vi "Calibration_Setup_file_2.0.vi"(2 "Data":T1={"Camera 1"={"Camera1"="", "Cam 1"=FALSE, "CAM1 Model"=enum."a2A5328-15ucBAS"}, "Camera 2"={"Camera2"="", "Cam 2"=FALSE, "CAM2 Model"=enum."a2A5328-15ucBAS"}, "Image"={"Camera1_Img"=refnum, "Camera2_Img"=refnum, "Img1_Orig_Disp"=refnum, "Img2_Orig_Disp"=refnum, "Img1_Orig_RGB"=refnum, "Img2_Orig_RGB"=refnum, "Blue_Plane_Extract"=refnum, "Subtracted_Plane"=refnum, "Img1_Binary"=refnum, "Img2_Binary"=refnum, "Crop_Mask"=refnum, "Img1_Save"=refnum, "Img2_Save"=refnum, "Img1_Cali_Full"=refnum, "Img2_Cali_Full"=refnum, "Img1_Cali_Detect"=refnum, "Img2_Cali_Detect"=refnum}, "Ques"={"Cam 1 queue"=refnum, "Cam 2 queue"=refnum, "Cam 1 - save queue"=refnum, "Cam 2 - save queue"=refnum, "Image Process Queue Size"=500, "Image Save Queue Size"=500, "Overload threshold"=500, "Max large object threshold"=0}, "Arduino SRS"={"Pinch-valve"="", "Actuator"=FALSE, "Open(T)/Close(F)"=FALSE}, "Pump"={"Pump"="", "Pump"=FALSE, "Pump State"=FALSE, "Pump Model"=enum."XLP6000", "Pump size"=FALSE, "Flush Size"=0, "Dispense Speed"=100, "Command"=""}, "Camera settings"={"Detection settings"={"Sample size threshold"=500, "Detection Region %"=30.0, "Timeout Sample"=200}, "Lens/camera settings"={"Aperture"=enum."Item 0", "Legacy Cam Attributes"=FALSE, "Max Framerate"=100, "Exposure Time"=1000.0, "Framerate"=15}, "Crop settings"={"Cam1"={"Rectangle 1"={"Left"=0, "Top"=0, "Right"=0, "Bottom"=0, "Rotation"=0.0}, "Camera Orientation 1"="", "Pixel to mm 1"=0.0}, "Cam2"={"Rectangle 2"={"Left"=0, "Top"=0, "Right"=0, "Bottom"=0, "Rotation"=0.0}, "Camera Orientation 2"="", "Pixel to mm 2"=0.0}}}, "Arduino ISS"={"Mega F3"="", "Phase3"=FALSE}, "Phase 3"={"Container nr."=0.0, "Mun. of containers"=0.0, "Size Interval"=0.0, "Initial size"=0.0, "Sorting sys."=FALSE, "Barcode"=""}, "Img_Capt"=FALSE, "Empty_Refill"=FALSE, "I don't think is in use"={"Crop"=FALSE, "Light intensity"=100, "Empty start"=1}, "Img_Capt Begin"=FALSE, "Extended setup"={"Location"="Station", "Latitude"="Station", "Longitude"="Station", "Determiner"="Station", "Sex"="Station", "Station"="", "Collection date"=""}, "Main interface"={"Sample Name"="Test Sample", "Operator"="JFR", "Species Name"="", "Other Notes"=""}, "Tap1"=0, "SystemVersion"=0, "System Serial"="", "Flush Insect"=FALSE, "Flush Error"=FALSE, "Start System"=FALSE, "Core JKI"={"Current VI Reference"=refnum, "Close Panel on Exit?"=FALSE}, "Calibration"={"Calibration 1"=path "C:/Users/au540322/Desktop/IHS_Project/images/Debris/Debris_0/Debris_0_2019_06_01-23-32-49-686.PNG", "Calibration 2"=path "C:/Users/au540322/Desktop/IHS_Project/images/Debris/Debris_0/Debris_0_2019_06_01-23-32-49-686.PNG", "Detect 1"=path "C:/Users/au540322/Desktop/IHS_Project/images/Debris/Debris_0/Debris_0_2019_06_01-23-32-49-686.PNG", "Detect 2"=path "C:/Users/au540322/Desktop/IHS_Project/images/Debris/Debris_0/Debris_0_2019_06_01-23-32-49-686.PNG"}} {"SystemVersion" items=["Standard", "XL"]; "Tap1" items=["Session Data", "Extended Setup", "Buffer", "Camera", "Dispenser", "Stats", "Connections"]; "I don't think is in use"."Empty start" min=1; "I don't think is in use"."Light intensity" scale=0.0..100.0; "Camera settings"."Crop settings"."Cam2"."Rectangle 2"."Rotation" format="%.2f"; "Camera settings"."Crop settings"."Cam2"."Rectangle 2"."Left" scale=0.0..1024.0; "Camera settings"."Crop settings"."Cam2"."Rectangle 2"."Right" scale=0.0..1024.0; "Camera settings"."Crop settings"."Cam1"."Rectangle 1"."Rotation" format="%.2f"; "Camera settings"."Crop settings"."Cam1"."Rectangle 1"."Left" scale=0.0..1024.0; "Camera settings"."Crop settings"."Cam1"."Rectangle 1"."Right" scale=0.0..1024.0; "Camera settings"."Lens/camera settings"."Framerate" min=1; "Camera settings"."Lens/camera settings"."Max Framerate" min=1; "Camera settings"."Detection settings"."Sample size threshold" min=1; "Pump"."Dispense Speed" min=1; "Pump"."Flush Size" min=0 max=6000 step=100; "Ques"."Overload threshold" min=1; "Ques"."Image Save Queue Size" min=1; "Ques"."Image Process Queue Size" min=1}, 3 "Path":string) -> ()   [LabVIEW 2024]
uses:
  controls/Data_JKI.ctl
  <vilib>/userDefined/High Color/IMAQdx.ctl
  <vilib>/vision/Image Controls.llb/IMAQ Image.ctl
  <vilib>/Utility/config.llb/Write Key (String).vi
  <vilib>/Utility/config.llb/NI_LVConfig.lvlib
panel:
  out "error out":errorcluster
  out "Error Out":errorcluster
  in  "Error In":errorcluster
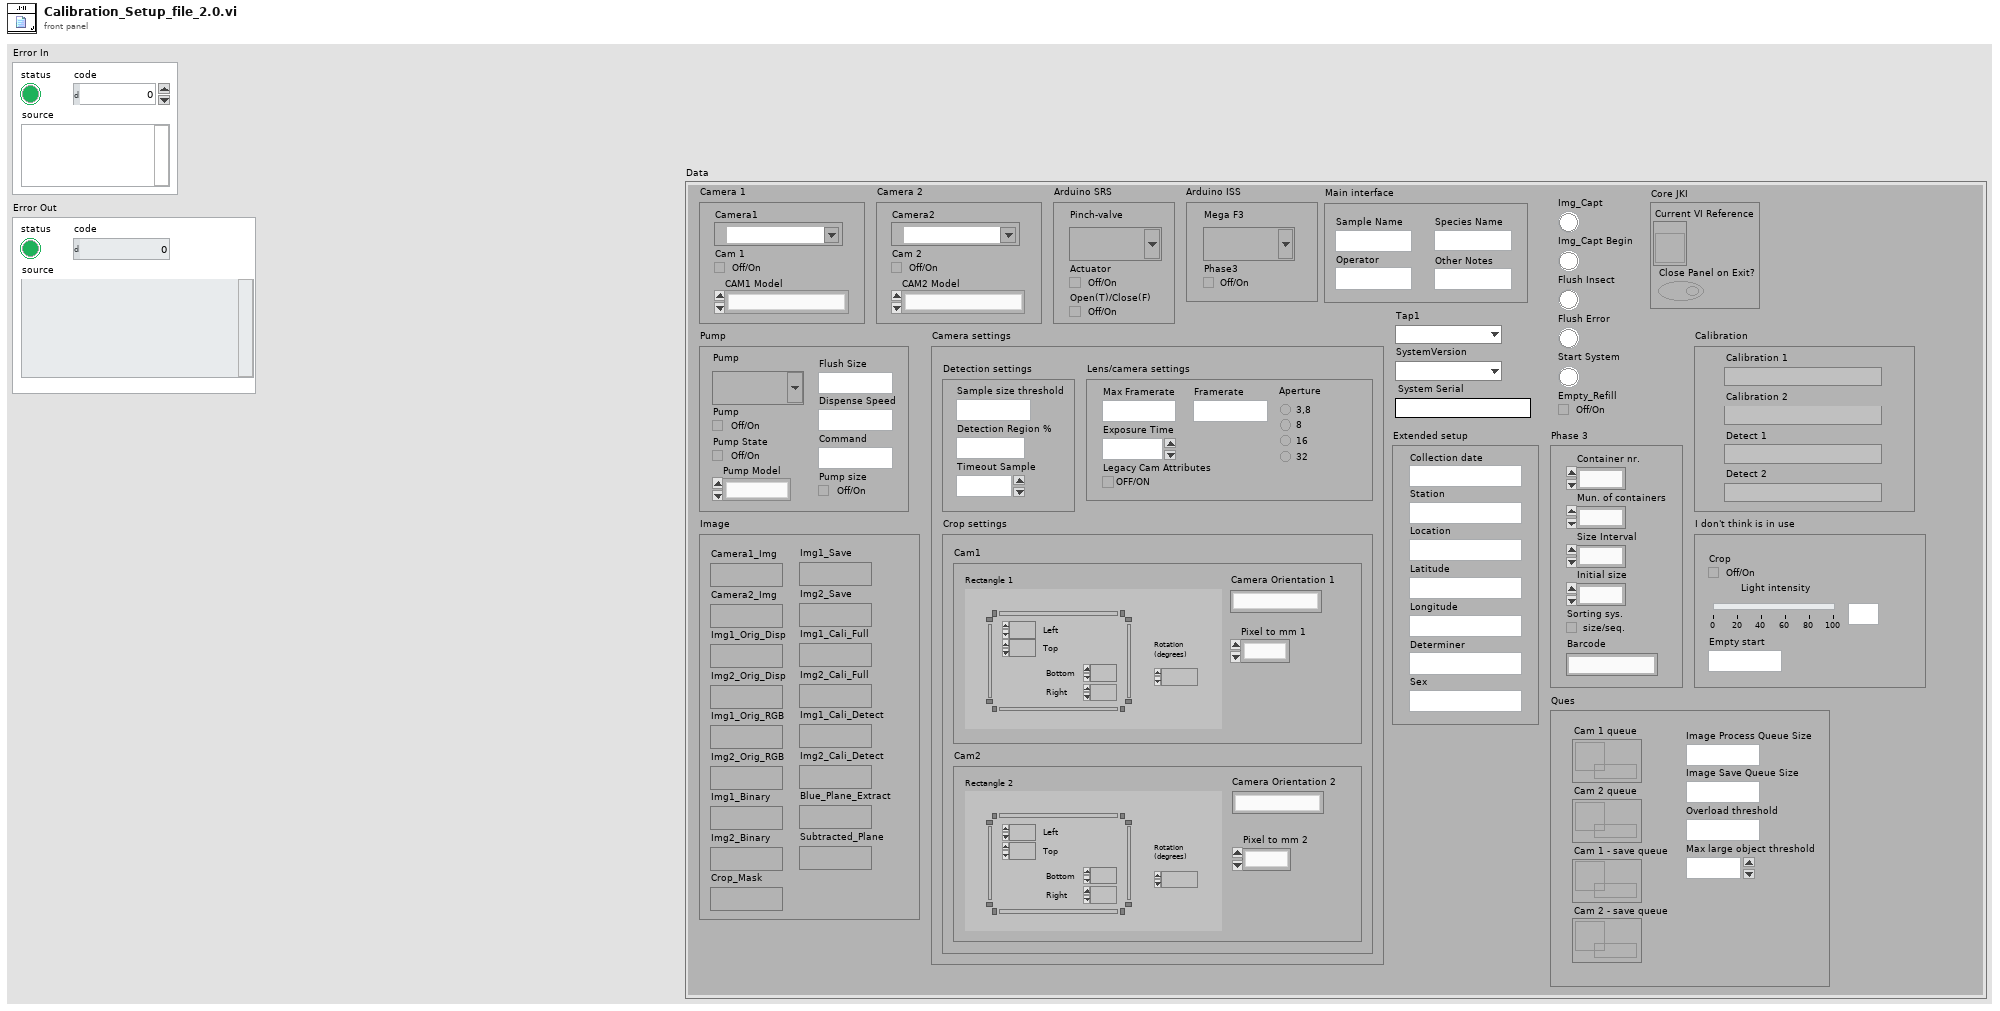
[diagram p1: front panel]
types:
  T1 = typedef "Data_JKI.ctl" = cluster{"Camera 1":cluster{"Camera1":T2, "Cam 1":bool, "CAM1 Model":enum16{"a2A5328-15ucBAS", "acA1920-155uc"}}, "Camera 2":cluster{"Camera2":T2, "Cam 2":bool, "CAM2 Model":enum16{"a2A5328-15ucBAS", "acA1920-155uc"}}, "Image":cluster{"Camera1_Img":T3, "Camera2_Img":T3, "Img1_Orig_Disp":T3, "Img2_Orig_Disp":T3, "Img1_Orig_RGB":T3, "Img2_Orig_RGB":T3, "Blue_Plane_Extract":T3, "Subtracted_Plane":T3, "Img1_Binary":T3, "Img2_Binary":T3, "Crop_Mask":T3, "Img1_Save":T3, "Img2_Save":T3, "Img1_Cali_Full":T3, "Img2_Cali_Full":T3, "Img1_Cali_Detect":T3, "Img2_Cali_Detect":T3}, "Ques":cluster{"Cam 1 queue":refnum<queue>, "Cam 2 queue":refnum<queue>, "Cam 1 - save queue":refnum<queue>, "Cam 2 - save queue":refnum<queue>, "Image Process Queue Size":i32, "Image Save Queue Size":i32, "Overload threshold":i32, "Max large object threshold":i32}, "Arduino SRS":cluster{"Pinch-valve":refnum<visa-resource-name>, "Actuator":bool, "Open(T)/Close(F)":bool}, "Pump":cluster{"Pump":refnum<visa-resource-name>, "Pump":bool, "Pump State":bool, "Pump Model":enum16{"XLP6000", "XL1000"}, "Pump size":bool, "Flush Size":i32, "Dispense Speed":i32, "Command":string}, "Camera settings":cluster{"Detection settings":cluster{"Sample size threshold":i32, "Detection Region %":dbl, "Timeout Sample":i32}, "Lens/camera settings":cluster{"Aperture":enum32{"Item 0", "Item 1", "Item 2", "Item 3"}, "Legacy Cam Attributes":bool, "Max Framerate":i32, "Exposure Time":dbl, "Framerate":i32}, "Crop settings":cluster{"Cam1":cluster{"Rectangle 1":T4, "Camera Orientation 1":string, "Pixel to mm 1":dbl}, "Cam2":cluster{"Rectangle 2":T4, "Camera Orientation 2":string, "Pixel to mm 2":dbl}}}, "Arduino ISS":cluster{"Mega F3":refnum<visa-resource-name>, "Phase3":bool}, "Phase 3":cluster{"Container nr.":dbl, "Mun. of containers":dbl, "Size Interval":dbl, "Initial size":dbl, "Sorting sys.":bool, "Barcode":string}, "Img_Capt":bool, "Empty_Refill":bool, "I don't think is in use":cluster{"Crop":bool, "Light intensity":i32, "Empty start":u32}, "Img_Capt Begin":bool, "Extended setup":cluster{"Location":string, "Latitude":string, "Longitude":string, "Determiner":string, "Sex":string, "Station":string, "Collection date":string}, "Main interface":cluster{"Sample Name":string, "Operator":string, "Species Name":string, "Other Notes":string}, "Tap1":u16, "SystemVersion":u16, "System Serial":string, "Flush Insect":bool, "Flush Error":bool, "Start System":bool, "Core JKI":cluster{"Current VI Reference":refnum<vi>, "Close Panel on Exit?":bool}, "Calibration":cluster{"Calibration 1":path, "Calibration 2":path, "Detect 1":path, "Detect 2":path}}
  T2 = typedef "IMAQdx.ctl" = refnum<k21>
  T3 = typedef "IMAQ Image.ctl" = refnum<image>
  T4 = typedef "IMAQ Rectangle" = cluster{"Left":i32, "Top":i32, "Right":i32, "Bottom":i32, "Rotation":dbl}
  T5 = typedef "NI_LVConfig.lvlib/Config Data RefNum.ctl" = refnum<k1>
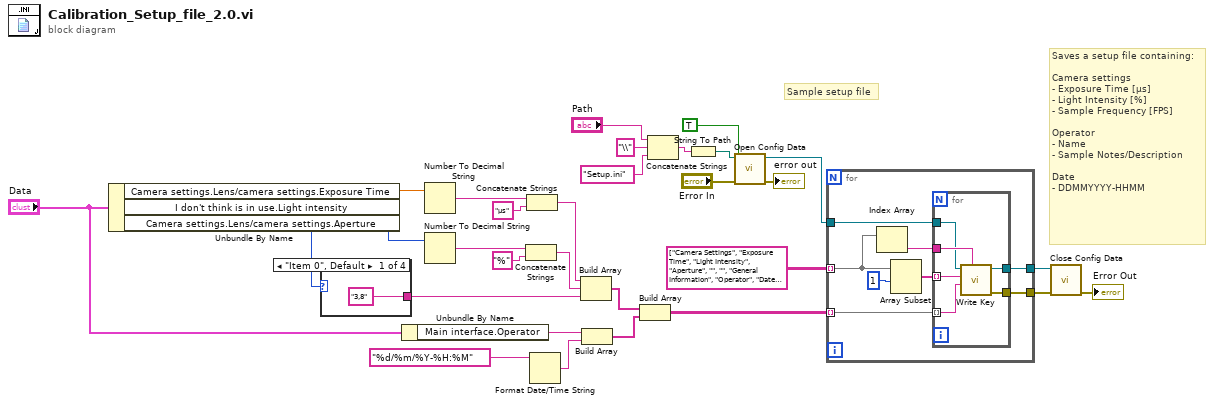
[diagram p0: block diagram]
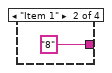
[diagram p2: hidden frame]
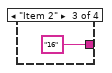
[diagram p3: hidden frame]
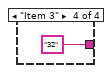
[diagram p4: hidden frame]
diagram:
  # "Saves a setup file containing:\n\nCamera settings\n- Exposure Time [µs]\n- Light Intensity [%]\n- Sample Frequency [FPS]\n\nOperator\n- Name\n- Sample Notes/Description\n\nDate\n- DDMMYYYY-HHMM"
  # "Sample setup file"
  n1 = Unbundle By Name("Data") -> ("Camera settings.Lens/camera settings.Exposure Time"=w20:dbl, "I don't think is in use.Light intensity"=w19:i32, "Camera settings.Lens/camera settings.Aperture"=w9:enum32{"Item 0", "Item 1", "Item 2", "Item 3"})
  n2 = case shown="\"Item 0\", Default" w9 {
    tunnel: ["3,8" "8" "16" "32"] -> w6
    frame "Item 0", Default {
    }
    frame "Item 1" {
    }
    frame "Item 2" {
    }
    frame "Item 3" {
    }
  }
  n3 = Unbundle By Name("Data") -> ("Main interface.Operator"=w10:string)
  n4 = Number To Decimal String(number=w20) -> (decimal integer string=w14:string)  [unwired: 1 in]
  n5 = Number To Decimal String(number=w19) -> (decimal integer string=w16:string)  [unwired: 1 in]
  n6 = Concatenate Strings(w16, "%" ("string")) -> (w15:string)
  n7 = Concatenate Strings(w14, "µs" ("string")) -> (w12:string)
  n8 = Format Date/Time String(time format string (%c)="%d/%m/%Y-%H:%M") -> (date/time string=w5:string)  [unwired: 2 in]
  n9 = Build Array(w12, w15, w6) -> (w30:string[])
  n10 = Build Array(w10, w5) -> (w11:string[])
  n11 = Build Array(w30, w11) -> (w29:string[][])
  n12 = Concatenate Strings("Path", "\\" ("string"), "Setup.ini" ("string")) -> (w23:string)
  n13 = String To Path(string=w23) -> (path=w25:path)
  n14 = call <vilib>:"Open Config Data.vi"("error in (no error)"="Error In", "create file if necessary (T)"=TRUE, "configuration file path"=w25) -> ("error out"=→"error out":errorcluster, "refnum"=w26:T5)  [unwired: 6 in, 1 out]
  n15 = for {
    tunnel: string[][] [["Camera Settings", "Exposure Time", "Light Intensity", "Aperture", "", ""], ["General Information", "Operator", "Date (DD/MM/YYYY)", "", "", ""], ["", "", "", "", "", ""]] ("appended array") -> [w41] mode=indexing
    tunnel: w29 -> [w39] mode=indexing
    tunnel: [w37] -> w28
    tunnel: [w36] -> w27
    tunnel: w26 -> [w35]
    n16 = Index Array(array=w41) -> (element=w40:string)  [unwired: 1 in]
    n17 = Array Subset(array=w41, index=1) -> (w38:string[])  [unwired: 1 in]
    n18 = for {
      tunnel: w40 -> [w48]
      tunnel: w39 -> [w47] mode=indexing
      tunnel: w38 -> [w46] mode=indexing
      tunnel: [w45] -> w37
      tunnel: [w44] -> w36
      tunnel: w35 -> [w43]
      n19 = call-poly <vilib>:"Write Key.vi"("section"=w48, "value"=w47, "key"=w46, "refnum"=w43) -> ("error out"=w44:errorcluster, "refnum out"=w45:T5)  [unwired: 5 in, 1 out]
    }
  }
  n20 = call <vilib>:"Close Config Data.vi"("error in (no error)"=w27, "refnum"=w28) -> ("error out"=→"Error Out":errorcluster)  [unwired: 8 in, 1 out]
